vi "CALC GEAR RATIO SPEEDS.vi"(8 "error in (no error)":errorcluster) -> (0 "error out":errorcluster, 1 "Vel ratios":T1, 2 "K LOADER":dbl format="%#_13g", 3 "K INTAKE":dbl format="%#_13g")   [LabVIEW 2023]
uses:
  ctrl defs/ctrl MOTOR SELECT.ctl
  Global INIT.vi
panel:
  out "SHOOTER MOTORS":T2 items=["REV NEO"=5676, "REV NEO 550"=11000, "VEX Falcon"=6380, "WC Kraken"=6000]
  out "SHOOTER ratio":dbl=4.0
  out "SHOOTER\n(rpm)":dbl
  out "R shooter (in)":dbl
  out "Vel SHOOTER\n(in/s) 2":dbl format="%_4f"
  out "INTAKE MOTOR":T2 items=["REV NEO"=5676, "REV NEO 550"=11000, "VEX Falcon"=6380, "WC Kraken"=6000]
  out "LOADER MOTORS":T2 items=["REV NEO"=5676, "REV NEO 550"=11000, "VEX Falcon"=6380, "WC Kraken"=6000]
  out "Vel LOADER\n(in/s)":dbl format="%_4f"
  out "R loader (in)":dbl
  out "LOADER\n(rpm)":dbl
  out "LOADER ratio":dbl=4.0
  out "INTAKE ratio":dbl=4.0
  out "R LG (in)":dbl format="%.3f"
  out "R SM (in)":dbl format="%.3f"
  out "large wheel\n(in/s)":dbl format="%_4f"
  out "small wheel\n(in/s)":dbl format="%_4f"
  out "INTAKE LG WHEEL\n(rpm)":dbl format="%#.3f"
  out "INTAKE SM WHEEL\n(rpm)":dbl format="%#.3f"
  out "INTAKE GEAR TRAIN\nGEAR RATIO\nto SM WHEEL":dbl
  out "INTAKE GEAR TRAIN\nGEAR RATIO\nto LRG WHEEL":dbl
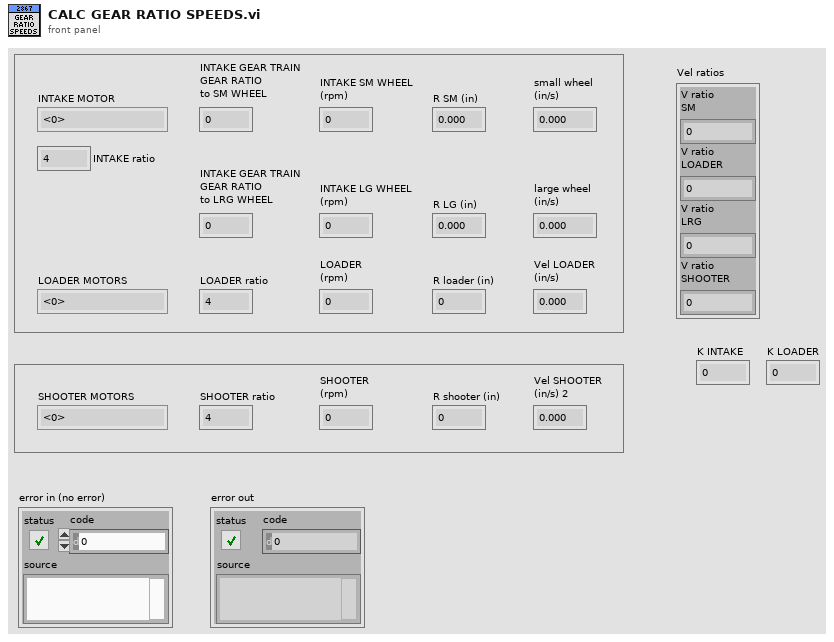
[diagram p1: front panel]
types:
  T1 = cluster{"V ratio\nSM":dbl, "V ratio\nLOADER":dbl, "V ratio\nLRG":dbl, "V ratio\nSHOOTER":dbl}
  T2 = typedef "ctrl MOTOR SELECT.ctl" = i16
  T3 = typedef "ctrl swerve motor.ctl" = cluster{"description":string, "MOTOR SELECT":T2, "Installed?":bool, "CAN ID":u8, "refnum name":string, "Invert":bool, "Idle Mode":T4, "Current limiting":T5, "MOTOR PIDF coefficients":T6, "gear ratio":dbl}
  T4 = typedef "Spark MAX Idle Mode.ctl" = enum16{"Coast", "Brake"}
  T5 = typedef "ctrl Spark MAX current limiting.ctl" = cluster{"Linearized":bool, "Free Speed (A)":dbl, "Primay (A)":dbl, "Limit RPM (0)":u32}
  T6 = typedef "ctrl motor PIDF coefficients.ctl" = cluster{"PIDF":cluster{"P Gain":dbl, "I Gain":dbl, "D Gain":dbl, "F Gain":dbl, "I Zone":dbl, "Min Output":dbl, "Max Output":dbl}, "Smart Motion":T7}
  T7 = typedef "Spark MAX Smart Motion Parameters.ctl" = cluster{"Max Velocity":dbl, "Max Acceleration":dbl, "Minimum Velocity Output":dbl, "Allowed Closed Loop Error":dbl}
  T8 = typedef "ctrl DEFINE GEAR.ctl" = cluster{"DP":dbl, "TEETH":i16, "DIAM (in)":dbl, "rev":bool, "ratio":dbl}
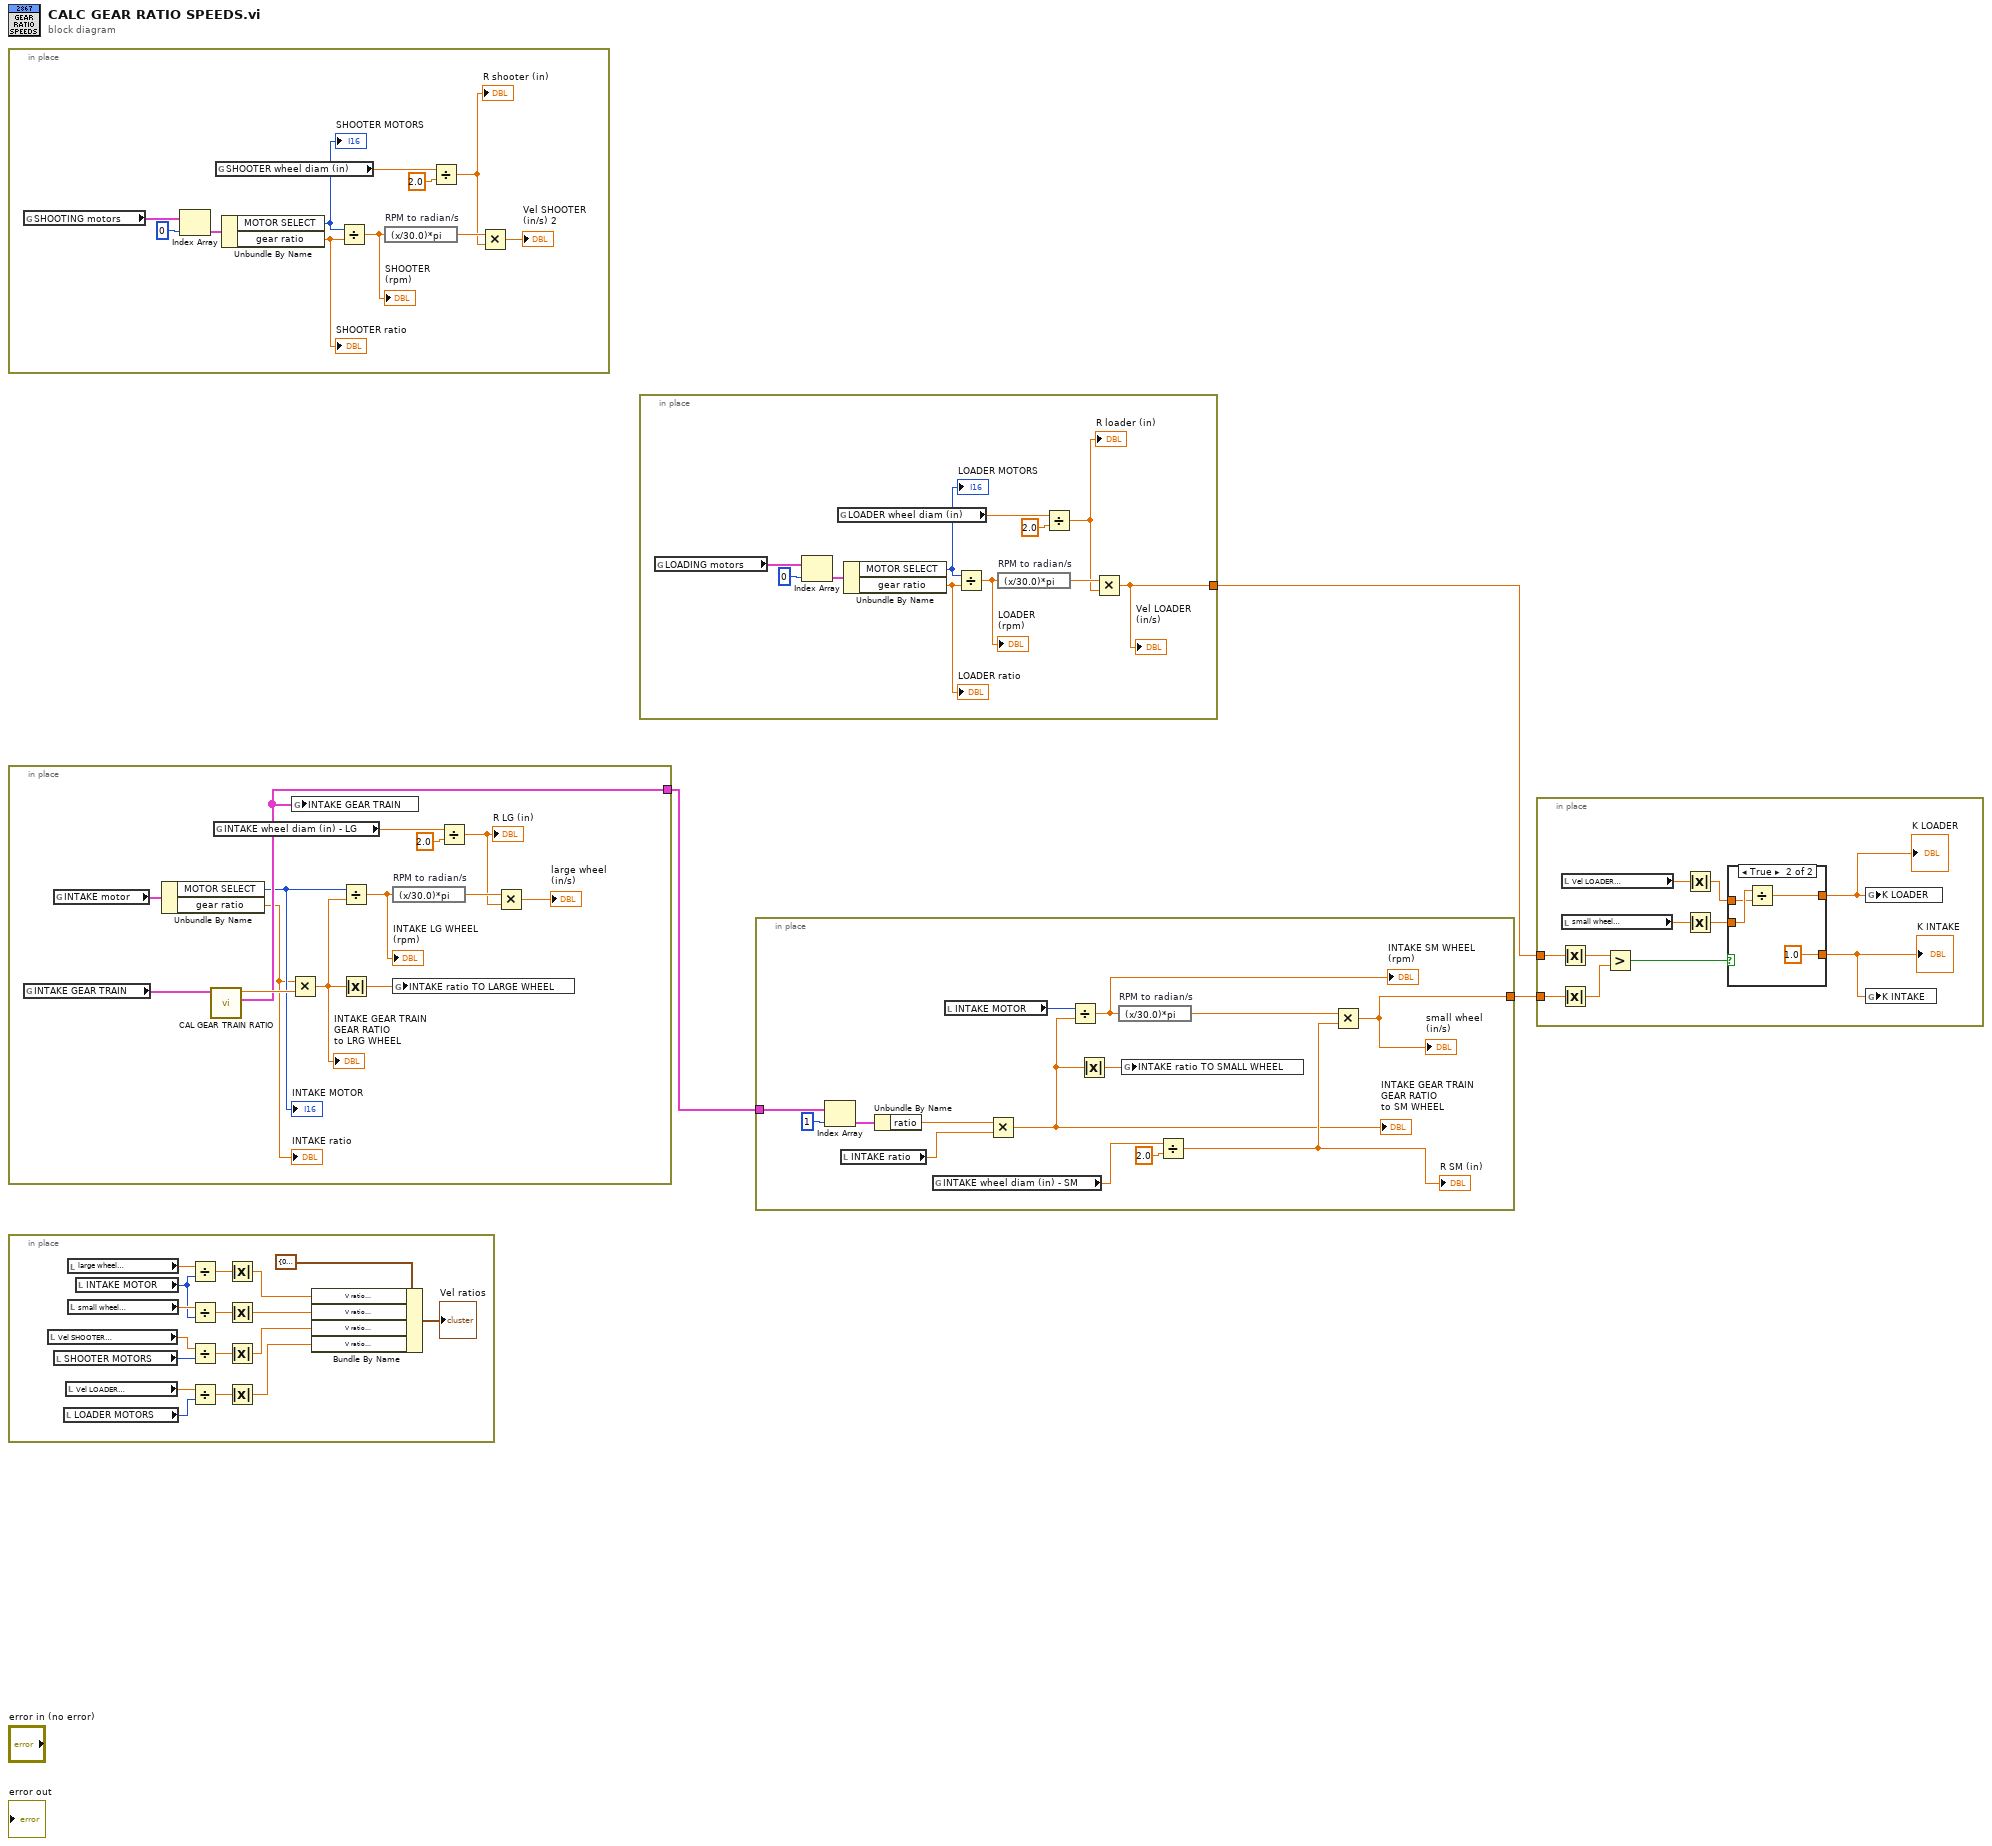
[diagram p0: block diagram]
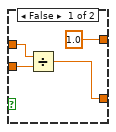
[diagram p2: hidden frame]
diagram:
  n1 = in-place {
    n2 = global read "Global INIT.vi" "SHOOTING motors"() -> (w8:T3[])
    n3 = Index Array(array=w8, index=0) -> (element=w6:T3)
    n4 = global read "Global INIT.vi" "SHOOTER wheel diam (in)"() -> (w14:dbl)
    n5 = Unbundle By Name(w6) -> ("MOTOR SELECT"=w5:T2, "gear ratio"=w4:dbl)
    "SHOOTER ratio" <- w4
    "SHOOTER MOTORS" <- w5
    n6 = Divide(x=w5, y=w4) -> (x/y=w12:dbl)
    "SHOOTER\n(rpm)" <- w12
    n7 = expression code="(x/30.0)*pi" "RPM to radian/s"(w12) -> (w11:dbl)
    n8 = Divide(x=w14, y=2.0) -> (x/y=w10:dbl)
    "R shooter (in)" <- w10
    n9 = Multiply(x=w11, y=w10) -> (x*y=→"Vel SHOOTER\n(in/s) 2":dbl)
  }
  n10 = in-place {
    in-place-border: [w20] -> w3
    n11 = global read "Global INIT.vi" "INTAKE GEAR TRAIN"() -> (w28:T8[])
    n12 = global read "Global INIT.vi" "INTAKE motor"() -> (w18:T3)
    n13 = Unbundle By Name(w18) -> ("MOTOR SELECT"=w17:T2, "gear ratio"=w15:dbl)
    "INTAKE MOTOR" <- w17
    "INTAKE ratio" <- w15
    n14 = call "CAL GEAR TRAIN RATIO.vi"("GEAR TRAIN definition"=w28) -> ("GEAR TRAIN updated"=w20:T8[], "GEAR RATIO"=w27:dbl)  [unwired: 9 in]
    n15 = global read "Global INIT.vi" "INTAKE wheel diam (in) - LG"() -> (w23:dbl)
    n16 = Multiply(x=w15, y=w27) -> (x*y=w19:dbl)
    "INTAKE GEAR TRAIN\nGEAR RATIO\nto LRG WHEEL" <- w19
    n17 = global write "Global INIT.vi" "INTAKE GEAR TRAIN"(w20) -> ()
    n18 = Divide(x=w17, y=w19) -> (x/y=w21:dbl)
    "INTAKE LG WHEEL\n(rpm)" <- w21
    n19 = Absolute Value(x=w19) -> (abs(x)=w16:dbl)
    n20 = expression code="(x/30.0)*pi" "RPM to radian/s"(w21) -> (w26:dbl)
    n21 = global write "Global INIT.vi" "INTAKE ratio TO LARGE WHEEL"(w16) -> ()
    n22 = Divide(x=w23, y=2.0) -> (x/y=w25:dbl)
    "R LG (in)" <- w25
    n23 = Multiply(x=w26, y=w25) -> (x*y=→"large wheel\n(in/s)":dbl)
  }
  n24 = in-place {
    n25 = local read "Vel SHOOTER\n(in/s) 2"() -> (w36:dbl)
    n26 = local read "SHOOTER MOTORS"() -> (w35:T2)
    n27 = local read "LOADER MOTORS"() -> (w43:T2)
    n28 = local read "Vel LOADER\n(in/s)"() -> (w44:dbl)
    n29 = local read "large wheel\n(in/s)"() -> (w38:dbl)
    n30 = local read "small wheel\n(in/s)"() -> (w45:dbl)
    n31 = local read "INTAKE MOTOR"() -> (w39:T2)
    n32 = Divide(x=w38, y=w39) -> (x/y=w40:dbl)
    n33 = Divide(x=w45, y=w39) -> (x/y=w42:dbl)
    n34 = Divide(x=w36, y=w35) -> (x/y=w37:dbl)
    n35 = Divide(x=w44, y=w43) -> (x/y=w41:dbl)
    n36 = Absolute Value(x=w40) -> (abs(x)=w32:dbl)
    n37 = Absolute Value(x=w42) -> (abs(x)=w31:dbl)
    n38 = Absolute Value(x=w37) -> (abs(x)=w30:dbl)
    n39 = Absolute Value(x=w41) -> (abs(x)=w29:dbl)
    n40 = Bundle By Name(cluster=T1 {"V ratio\nSM"=0.026179938779914945, "V ratio\nLOADER"=0.03599741582238305, "V ratio\nLRG"=0.05235987755982989, "V ratio\nSHOOTER"=0.05235987755982989} ("Cluster"), "V ratio\nLRG"=w32, "V ratio\nSM"=w31, "V ratio\nSHOOTER"=w30, "V ratio\nLOADER"=w29) -> (→"Vel ratios":T1)
  }
  n41 = in-place {
    in-place-border: [w47] -> w2
    n42 = global read "Global INIT.vi" "LOADING motors"() -> (w50:T3[])
    n43 = Index Array(array=w50, index=0) -> (element=w51:T3)
    n44 = global read "Global INIT.vi" "LOADER wheel diam (in)"() -> (w56:dbl)
    n45 = Unbundle By Name(w51) -> ("MOTOR SELECT"=w48:T2, "gear ratio"=w46:dbl)
    "LOADER ratio" <- w46
    "LOADER MOTORS" <- w48
    n46 = Divide(x=w48, y=w46) -> (x/y=w54:dbl)
    "LOADER\n(rpm)" <- w54
    n47 = expression code="(x/30.0)*pi" "RPM to radian/s"(w54) -> (w53:dbl)
    n48 = Divide(x=w56, y=2.0) -> (x/y=w52:dbl)
    "R loader (in)" <- w52
    n49 = Multiply(x=w53, y=w52) -> (x*y=w47:dbl)
    "Vel LOADER\n(in/s)" <- w47
  }
  n50 = in-place {
    in-place-border: w3 -> [w65]
    in-place-border: [w59] -> w1
    n51 = Index Array(array=w65, index=1) -> (element=w63:T8)
    n52 = local read "INTAKE ratio"() -> (w61:dbl)
    n53 = Unbundle By Name(w63) -> ("ratio"=w60:dbl)
    n54 = global read "Global INIT.vi" "INTAKE wheel diam (in) - SM"() -> (w69:dbl)
    n55 = local read "INTAKE MOTOR"() -> (w58:T2)
    n56 = Multiply(x=w60, y=w61) -> (x*y=w62:dbl)
    "INTAKE GEAR TRAIN\nGEAR RATIO\nto SM WHEEL" <- w62
    n57 = Divide(x=w58, y=w62) -> (x/y=w70:dbl)
    "INTAKE SM WHEEL\n(rpm)" <- w70
    n58 = Absolute Value(x=w62) -> (abs(x)=w57:dbl)
    n59 = expression code="(x/30.0)*pi" "RPM to radian/s"(w70) -> (w67:dbl)
    n60 = global write "Global INIT.vi" "INTAKE ratio TO SMALL WHEEL"(w57) -> ()
    n61 = Divide(x=w69, y=2.0) -> (x/y=w66:dbl)
    "R SM (in)" <- w66
    n62 = Multiply(x=w67, y=w66) -> (x*y=w59:dbl)
    "small wheel\n(in/s)" <- w59
  }
  n63 = in-place {
    in-place-border: w2 -> [w80]
    in-place-border: w1 -> [w79]
    n64 = Absolute Value(x=w80) -> (abs(x)=w76:dbl)
    n65 = Absolute Value(x=w79) -> (abs(x)=w75:dbl)
    n66 = local read "Vel LOADER\n(in/s)"() -> (w78:dbl)
    n67 = local read "small wheel\n(in/s)"() -> (w77:dbl)
    n68 = Greater?(x=w76, y=w75) -> (0:w81:bool)
    n69 = Absolute Value(x=w78) -> (abs(x)=w74:dbl)
    n70 = Absolute Value(x=w77) -> (abs(x)=w73:dbl)
    n71 = case shown="True" w81 {
      tunnel: w74 -> [w83 w86]
      tunnel: [1.0 w89] -> w72
      tunnel: [w84 1.0] -> w71
      tunnel: w73 -> [w82 w87]
      frame False {
        n72 = Divide(x=w83, y=w82) -> (x/y=w84:dbl)
      }
      frame True {
        n73 = Divide(x=w87, y=w86) -> (x/y=w89:dbl)
      }
    }
    "K INTAKE" <- w71
    "K LOADER" <- w72
    n74 = global write "Global INIT.vi" "K LOADER"(w72) -> ()
    n75 = global write "Global INIT.vi" "K INTAKE"(w71) -> ()
  }
